vi "start_ThreadPool.vi"(0 "Host_Reference":refnum<class "HGF_Reference.lvclass">, 2 "timeout in ms (-1)":i32, 5 "error in (no error)":errorcluster) -> (14 "dup Host_Reference":refnum<class "HGF_Reference.lvclass">, 16 "dup timeout in ms":i32, 17 "HGF_ThreadPool_Reference":refnum<class "HGF_Reference.lvclass">, 19 "error out":errorcluster)   [LabVIEW 2009, in "MoAgSy.lvlib" / "MoAgSy_Host.lvclass"]
doc: "<B>public</B> VI starts a threadpool and creates a threadpool reference. The threadpool is needed to manage the agent systems engines.\n<B>Error handling and error retry not yet implemented</B>\n\nF.Berck@gsi.de\nGSI Darmstadt 2009"
uses:
  MoAgSy_Host.lvclass
  HGF_BaseClasses/HGF_Reference/HGF_Reference.lvclass
  HGF_BaseClasses/HGF_Factory/HGF_Factory.lvclass
  HGF_BaseClasses/HGF_ThreadPool/HGF_ThreadPool.lvclass
  MoAgSy.lvlib
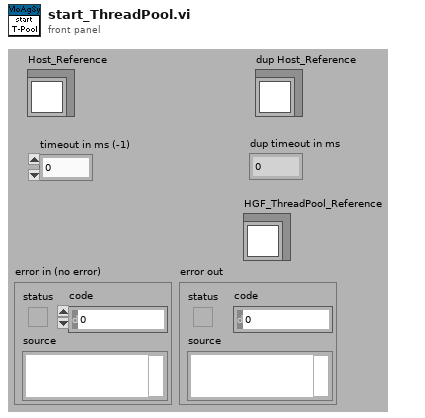
[diagram p1: front panel]
types:
  T1 = cluster{"Host Name":string, "Maximum number of running Agents":i16, "ID":string}
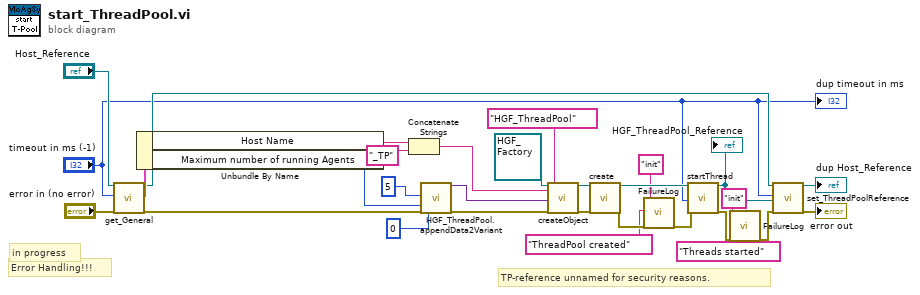
[diagram p0: block diagram]
diagram:
  # "TP-reference unnamed for security reasons."
  # "Error Handling!!!"
  # "in progress"
  n1 = call "get_General.vi"("Host_Reference"="Host_Reference", "timeout in ms (-1)"="timeout in ms (-1)", "error in (no error)"="error in (no error)") -> ("dup Host_Reference"=w18:refnum<class "HGF_Reference.lvclass">, "General"=w25:T1, "error out"=w30:errorcluster)  [unwired: 14 out]
  n2 = Unbundle By Name(w25) -> ("Host Name"=w11:string, "Maximum number of running Agents"=w10:i16)
  n3 = Concatenate Strings(w11, "_TP" ("string")) -> (w16:string)
  n4 = call "HGF_ThreadPool.appendData2Variant.vi"("initialNofThreads (0)"=5, "maxNofThreads (-1:unlimited)"=w10, "error in (no error)"=w30, "autoIncrementLimit (-1)"=0) -> ("dup initData"=w29:variant, "error out"=w22:errorcluster)  [unwired: 3 in, 11 out]
  n5 = call "createObject.vi"("HGF_Factory"=refnum<class "HGF_Factory.lvclass"> refnum ("HGF_BaseClasses.lvlib:HGF_Factory.lvclass"), "objectName"=w16, "initializationData"=w29, "error in (no error)"=w22, "className"="HGF_ThreadPool") -> ("HGF_Object"=w21:refnum<class "HGF_Factory.lvclass">, "error out"=w19:errorcluster)  [unwired: 13 out]
  n6 = call "create.vi"("Object"=w21, "error in (no error)"=w19) -> ("HGF_Reference"=w20:refnum<class "HGF_Reference.lvclass">, "error out"=w8:errorcluster)  [unwired: 1 in, 15 out]
  n7 = call "FailureLog.vi"("Section"="init", "key"="ThreadPool created", "error in (no error)"=w8) -> ("error out"=w7:errorcluster)  [unwired: 16 in]
  n8 = call "startThread.vi"("HGF_ThreadPool_Reference"=w20, "timeout in ms (-1)"="timeout in ms (-1)", "error in (no error)"=w7) -> ("dup HGF_ThreadPool_Reference"=w15:refnum<class "HGF_Reference.lvclass">, "error out"=w4:errorcluster)  [unwired: 15 out]
  "HGF_ThreadPool_Reference" <- w15
  n9 = call "FailureLog.vi"("Section"="init", "key"="Threads started", "error in (no error)"=w4) -> ("error out"=w3:errorcluster)  [unwired: 16 in]
  n10 = call "set_ThreadPoolReference.vi"("Host_Reference"=w18, "timeout in ms (-1)"="timeout in ms (-1)", "Threadpool Reference"=w15, "error in (no error)"=w3) -> ("dup Host_Reference"=→"dup Host_Reference":refnum<class "HGF_Reference.lvclass">, "error out"=→"error out":errorcluster)  [unwired: 14 out]
  "dup timeout in ms" <- "timeout in ms (-1)"
